vi "Disabled.vi"(7 "Robot Mode":T2, 10 "Match Info":T1={"Autonomous Elapsed Seconds"=0.0, "TeleOp Elapsed Seconds"=0.0, "Disabled Elapsed Seconds"=0.0, "Visited Autonomous"=FALSE, "Visited TeleOp"=FALSE, "Visited Disabled"=FALSE, "Autonomous Settings"={"Autonomous Style"=enum."Independent", "VI Refnum"=refnum}}, 11 "Call Context":T3) -> ()   [LabVIEW 2012]
doc: "This VI is called each time a disabled packet is received from the DS. It is often used to prepare for the next robot mode, to calibrate sensors, etc."
uses:
  <vilib>/Rock Robotics/WPI/DriverStation/WPI_DriverStationDerivedRobotMode.ctl
  <vilib>/Rock Robotics/WPI/DriverStation/WPI_DriverStationRobotMode2.ctl
  <vilib>/Rock Robotics/WPI/DriverStation/WPI_DriverStationMatch Info.ctl
  Robot Global Data.vi
  <vilib>/Rock Robotics/WPI/Joystick/WPI_JoystickGetSetRefNum.vi
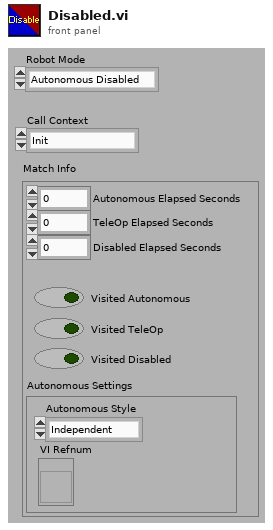
[diagram p1: front panel]
types:
  T1 = typedef "WPI_DriverStationMatch Info.ctl" = cluster{"Autonomous Elapsed Seconds":dbl, "TeleOp Elapsed Seconds":dbl, "Disabled Elapsed Seconds":dbl, "Visited Autonomous":bool, "Visited TeleOp":bool, "Visited Disabled":bool, "Autonomous Settings":cluster{"Autonomous Style":enum16{"Iterative", "Independent"}, "VI Refnum":refnum<vi>}}
  T2 = typedef "WPI_DriverStationRobotMode2.ctl" = enum16{"Autonomous Disabled", "Autonomous Enabled", "Teleop Disabled", "Teleop Enabled", "Timeout", "Finish", "Test Disabled", "Test Enabled"}
  T3 = typedef "WPI_DriverStationDerivedRobotMode.ctl" = enum16{"Init", "Execute", "Stop"}
  T4 = typedef "WPI_JoystickDevRef.ctl" = cluster{"Device":T5}
  T5 = typedef "WPI_JoystickDeviceEnum.ctl" = enum16{"USB 1", "USB 2", "USB 3", "USB 4", "Kinect 1", "Kinect 2"}
  T6 = typedef "WPI_JoystickButtonState.ctl" = cluster{"Button 1":bool, "Button 2":bool, "Button 3":bool, "Button 4":bool, "Button 5":bool, "Button 6":bool, "Button 7":bool, "Button 8":bool, "Button 9":bool, "Button 10":bool, "Button 11":bool, "Button 12":bool}
  T7 = cluster{"Setpoint 1":dbl, "Setpoint 2":dbl, "Setpoint 3":dbl, "Setpoint 4":dbl, "RotLow":dbl, "RotHigh":dbl, "ExtLow":dbl, "ExtHigh":dbl}
  T8 = cluster{"FlipperLeftUp":dbl, "FlipperLeftDown":dbl, "FlipperRightUp":dbl, "FlipperRightDown":dbl, "KickerLeftBack":dbl, "KickerLeftForward":dbl, "KickerRightBack":dbl, "KickerRightForward":dbl}
  T9 = typedef "WPI_MotorControlDeviceRef.ctl" = cluster{"DeviceStatus":errorcluster, "Type":enum16{"PWM", "CAN"}, "PWM":cluster{"Digital Module":T10, "PWM Channel":T11, "DeadBand":T12}, "CAN":cluster{"Device Number":u8, "Control Mode":T13, "Semaphore":T14, "Max Vout":dbl}, "Invert":bool, "TransformRef":T15, "InvTransformRef":T15}
  T10 = typedef "FPGA_TypedefDigitalModule.ctl" = enum16{"Digital Module 1", "Digital Module 2"}
  T11 = typedef "FPGA_DIOPWMChannel.ctl" = enum8{"PWM 1", "PWM 2", "PWM 3", "PWM 4", "PWM 5", "PWM 6", "PWM 7", "PWM 8", "PWM 9", "PWM 10", "Invalid"}
  T12 = typedef "WPI_PWMDeadband.ctl" = cluster{"Name":string, "maxPositivePwm":i32, "minPositivePwm":i32, "centerPwm":i32, "maxNegativePwm":i32, "minNegativePwm":i32, "angularRange":u16}
  T13 = typedef "WPI_CANJaguar_ControlMode.ctl" = enum8{"Percent VBus", "Current", "Speed", "Position", "Voltage"}
  T14 = typedef "Semaphore RefNum" = refnum<k1>
  T15 = typedef "WPI_PWMTransform_ConPane.ctl" = refnum<vi>
  T16 = typedef "WPI_ServoDeviceRef.ctl" = cluster{"DeviceStatus":errorcluster, "Digital Module":T10, "PWM Channel":T11, "DeadBand":T12}
  T17 = cluster{"Right Servo High":dbl, "Right Servo Mid":dbl, "Right Servo Low":dbl, "Left Servo High":dbl, "Left Servo Mid":dbl, "Left Servo Low":dbl}
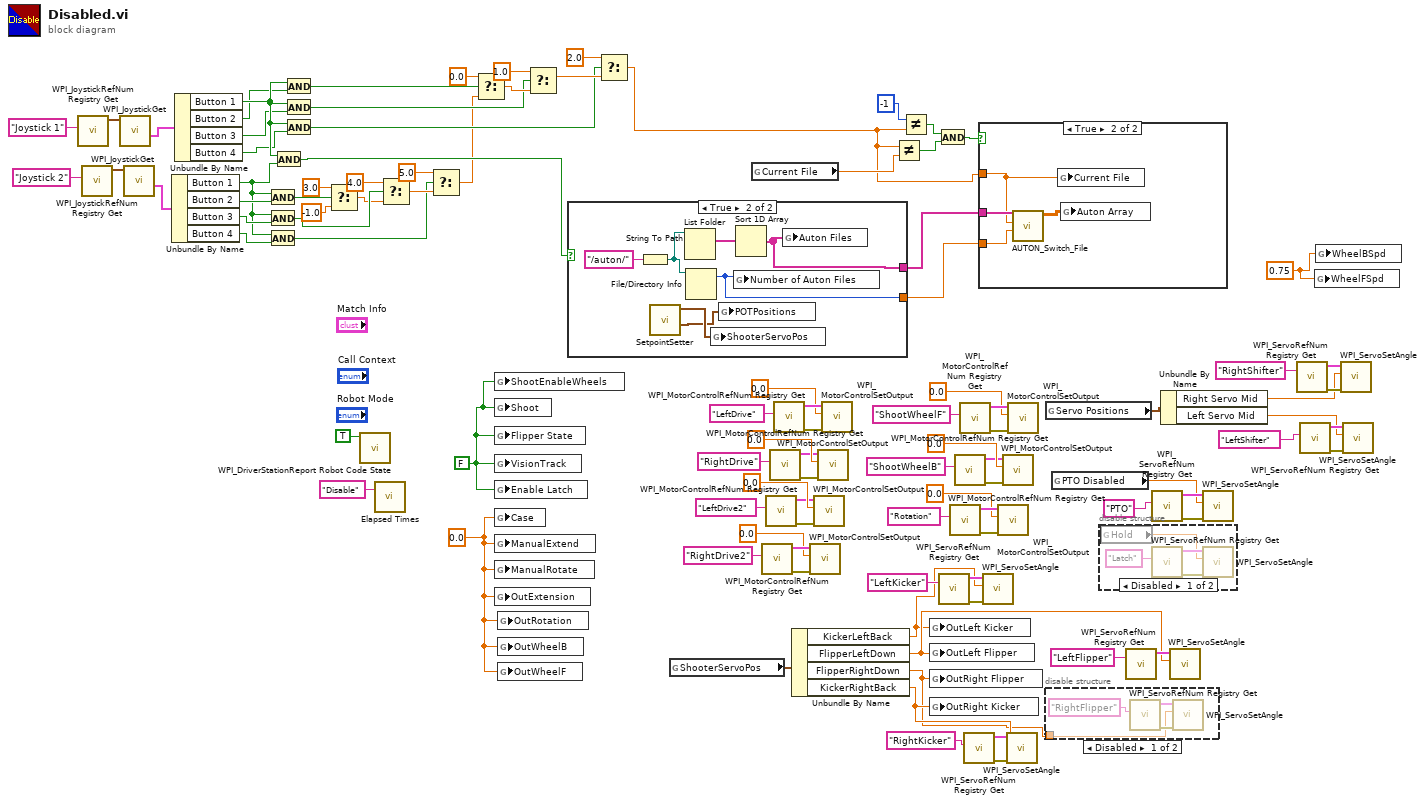
[diagram p0: block diagram]
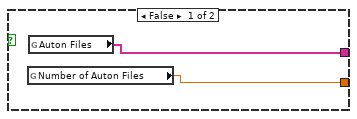
[diagram p5: hidden frame]
diagram:
  w35 = 0.75 ("Case")
  w54 = 0.0 ("Case")
  w55 = FALSE ("Enable Latch")
  n1 = call <vilib>:"WPI_JoystickRefNum Registry Get.vi"("refnum name"="Joystick 1") -> ("JoystickDevRef"=w33:T4)  [unwired: 9 in, 1 out]
  n2 = call <vilib>:"WPI_JoystickRefNum Registry Get.vi"("refnum name"="Joystick 2") -> ("JoystickDevRef"=w31:T4)  [unwired: 9 in, 1 out]
  n3 = call <vilib>:"WPI_JoystickGet.vi"("JoystickDevRef"=w33) -> ("Buttons"=w29:T6)  [unwired: 4 in, 2 out]
  n4 = call <vilib>:"WPI_JoystickGet.vi"("JoystickDevRef"=w31) -> ("Buttons"=w30:T6)  [unwired: 4 in, 2 out]
  n5 = Unbundle By Name(w30) -> ("Button 1"=w26:bool, "Button 2"=w28:bool, "Button 3"=w27:bool, "Button 4"=w25:bool)
  n6 = Unbundle By Name(w29) -> ("Button 1"=w7:bool, "Button 2"=w6:bool, "Button 3"=w5:bool, "Button 4"=w4:bool)
  n7 = And(x=w26, y=w28) -> (x .and. y?=w24:bool)
  n8 = And(x=w26, y=w27) -> (x .and. y?=w21:bool)
  n9 = And(x=w26, y=w25) -> (x .and. y?=w15:bool)
  n10 = And(x=w7, y=w26) -> (x .and. y?=w17:bool)
  n11 = And(x=w7, y=w6) -> (x .and. y?=w8:bool)
  n12 = And(x=w7, y=w5) -> (x .and. y?=w10:bool)
  n13 = And(x=w7, y=w4) -> (x .and. y?=w3:bool)
  n14 = Select(t=3.0, s=w24, f=-1.0) -> (s? t:f=w20:dbl)
  n15 = call <vilib>:"WPI_DriverStationReport Robot Code State.vi"("Disabled"=TRUE ("Autonomous")) -> ()  [unwired: 10 in, 1 out]
  n16 = call "Elapsed Times.vi"("Call Name"="Disable") -> ()  [unwired: 2 in, 1 out]
  n17 = Select(t=4.0, s=w21, f=w20) -> (s? t:f=w18:dbl)
  n18 = Select(t=5.0, s=w15, f=w18) -> (s? t:f=w2:dbl)
  n19 = Select(t=0.0, s=w8, f=w2) -> (s? t:f=w11:dbl)
  n20 = global write "Robot Global Data.vi" "ShootEnableWheels"(w55) -> ()
  n21 = global write "Robot Global Data.vi" "Shoot"(w55) -> ()
  n22 = global write "Robot Global Data.vi" "Flipper State"(w55) -> ()
  n23 = global write "Robot Global Data.vi" "VisionTrack"(w55) -> ()
  n24 = global write "Robot Global Data.vi" "Enable Latch"(w55) -> ()
  n25 = global write "Robot Global Data.vi" "Case"(w54) -> ()
  n26 = global write "Robot Global Data.vi" "ManualExtend"(w54) -> ()
  n27 = global write "Robot Global Data.vi" "ManualRotate"(w54) -> ()
  n28 = global write "Robot Global Data.vi" "OutExtension"(w54) -> ()
  n29 = global write "Robot Global Data.vi" "OutRotation"(w54) -> ()
  n30 = global write "Robot Global Data.vi" "OutWheelB"(w54) -> ()
  n31 = global write "Robot Global Data.vi" "OutWheelF"(w54) -> ()
  n32 = Select(t=1.0, s=w10, f=w11) -> (s? t:f=w13:dbl)
  n33 = case shown="True" w17 {
    tunnel: [w101 w106] -> w90
    tunnel: [w102 w105] -> w85
    frame False {
      n34 = global read "Robot Global Data.vi" "Number of Auton Files"() -> (w101:dbl)
      n35 = global read "Robot Global Data.vi" "Auton Files"() -> (w102:string[])
    }
    frame True {
      n36 = String To Path(string="/auton/") -> (path=w108:path)
      n37 = call "SetpointSetter.vi"() -> ("Arm Pos"=w103:T7, "Shooter Servo Pos"=w104:T8)  [unwired: 10 in]
      n38 = List Folder(path=w108) -> (filenames=w107:string[])  [unwired: 3 in, 3 out]
      n39 = File/Directory Info(path=w108) -> (size=w106:i64)  [unwired: 1 in, 6 out]
      n40 = global write "Robot Global Data.vi" "ShooterServoPos"(w104) -> ()
      n41 = global write "Robot Global Data.vi" "POTPositions"(w103) -> ()
      n42 = global write "Robot Global Data.vi" "Number of Auton Files"(w106) -> ()
      n43 = Sort 1D Array(array=w107) -> (sorted array=w105:string[])
      n44 = global write "Robot Global Data.vi" "Auton Files"(w105) -> ()
    }
  }
  n45 = Select(t=2.0, s=w3, f=w13) -> (s? t:f=w1:dbl)
  n46 = global read "Robot Global Data.vi" "ShooterServoPos"() -> (w53:T8)
  n47 = global read "Robot Global Data.vi" "Current File"() -> (w88:dbl)
  n48 = call <vilib>:"WPI_MotorControlRefNum Registry Get.vi"("refnum name"="RightDrive2") -> ("error out"=w71:errorcluster, "MotorControlDevRef"=w70:T9)  [unwired: 9 in]
  n49 = call <vilib>:"WPI_MotorControlRefNum Registry Get.vi"("refnum name"="LeftDrive2") -> ("error out"=w64:errorcluster, "MotorControlDevRef"=w65:T9)  [unwired: 9 in]
  n50 = call <vilib>:"WPI_MotorControlRefNum Registry Get.vi"("refnum name"="RightDrive") -> ("error out"=w91:errorcluster, "MotorControlDevRef"=w92:T9)  [unwired: 9 in]
  n51 = call <vilib>:"WPI_MotorControlRefNum Registry Get.vi"("refnum name"="LeftDrive") -> ("error out"=w98:errorcluster, "MotorControlDevRef"=w97:T9)  [unwired: 9 in]
  n52 = Unbundle By Name(w53) -> ("KickerLeftBack"=w50:dbl, "FlipperLeftDown"=w51:dbl, "FlipperRightDown"=w49:dbl, "KickerRightBack"=w52:dbl)
  n53 = call <vilib>:"WPI_MotorControlSetOutput.vi"("error in (no error)"=w71, "Output"=0.0, "MotorControlDevRef"=w70) -> ()  [unwired: 6 in, 3 out]
  n54 = call <vilib>:"WPI_MotorControlSetOutput.vi"("error in (no error)"=w64, "Output"=0.0, "MotorControlDevRef"=w65) -> ()  [unwired: 6 in, 3 out]
  n55 = call <vilib>:"WPI_MotorControlSetOutput.vi"("error in (no error)"=w91, "Output"=0.0, "MotorControlDevRef"=w92) -> ()  [unwired: 6 in, 3 out]
  n56 = call <vilib>:"WPI_MotorControlSetOutput.vi"("error in (no error)"=w98, "Output"=0.0, "MotorControlDevRef"=w97) -> ()  [unwired: 6 in, 3 out]
  n57 = Not Equal?(x=w1, y=w88) -> (x != y?=w86:bool)
  n58 = Not Equal?(x=-1, y=w1) -> (x != y?=w87:bool)
  n59 = global write "Robot Global Data.vi" "OutLeft Kicker"(w50) -> ()
  n60 = global write "Robot Global Data.vi" "OutLeft Flipper"(w51) -> ()
  n61 = global write "Robot Global Data.vi" "OutRight Flipper"(w49) -> ()
  n62 = global write "Robot Global Data.vi" "OutRight Kicker"(w52) -> ()
  n63 = And(x=w87, y=w86) -> (x .and. y?=w84:bool)
  n64 = call <vilib>:"WPI_ServoRefNum Registry Get.vi"("refnum name"="LeftKicker") -> ("error out"=w56:errorcluster, "ServoDeviceRef"=w57:T16)  [unwired: 9 in]
  n65 = call <vilib>:"WPI_MotorControlRefNum Registry Get.vi"("refnum name"="Rotation") -> ("error out"=w75:errorcluster, "MotorControlDevRef"=w74:T9)  [unwired: 9 in]
  n66 = call <vilib>:"WPI_MotorControlRefNum Registry Get.vi"("refnum name"="ShootWheelB") -> ("error out"=w76:errorcluster, "MotorControlDevRef"=w77:T9)  [unwired: 9 in]
  n67 = call <vilib>:"WPI_MotorControlRefNum Registry Get.vi"("refnum name"="ShootWheelF") -> ("error out"=w83:errorcluster, "MotorControlDevRef"=w82:T9)  [unwired: 9 in]
  n68 = call <vilib>:"WPI_ServoRefNum Registry Get.vi"("refnum name"="RightKicker") -> ("error out"=w62:errorcluster, "ServoDeviceRef"=w60:T16)  [unwired: 9 in]
  n69 = case shown="True" w84 {
    tunnel: w85 -> [_ w113]
    tunnel: w90 -> [_ w112]
    tunnel: w1 -> [_ w110]
    frame False {
    }
    frame True {
      n70 = call "AUTON_Switch_File.vi"("Number of Auton Files"=w112, "Auton File"=w110, "Auton Files"=w113) -> ("Auton Array"=w111:dbl[][])  [unwired: 7 in, 1 out]
      n71 = global write "Robot Global Data.vi" "Current File"(w110) -> ()
      n72 = global write "Robot Global Data.vi" "Auton Array"(w111) -> ()
    }
  }
  n73 = call <vilib>:"WPI_ServoSetAngle.vi"("error in (no error)"=w56, "Angle"=w50, "ServoDeviceRef"=w57) -> ()  [unwired: 7 in, 2 out]
  n74 = call <vilib>:"WPI_MotorControlSetOutput.vi"("error in (no error)"=w75, "Output"=0.0, "MotorControlDevRef"=w74) -> ()  [unwired: 6 in, 3 out]
  n75 = call <vilib>:"WPI_MotorControlSetOutput.vi"("error in (no error)"=w76, "Output"=0.0, "MotorControlDevRef"=w77) -> ()  [unwired: 6 in, 3 out]
  n76 = call <vilib>:"WPI_ServoSetAngle.vi"("error in (no error)"=w62, "Angle"=w52, "ServoDeviceRef"=w60) -> ()  [unwired: 7 in, 2 out]
  n77 = call <vilib>:"WPI_MotorControlSetOutput.vi"("error in (no error)"=w83, "Output"=0.0, "MotorControlDevRef"=w82) -> ()  [unwired: 6 in, 3 out]
  n78 = global read "Robot Global Data.vi" "Servo Positions"() -> (w39:T17)
  n79 = disable-structure shown="Disabled" {
    disable-tunnel: w49 -> [w114 _]
    frame Disabled {
      n80 = call <vilib>:"WPI_ServoRefNum Registry Get.vi"("refnum name"="RightFlipper") -> ("error out"=w117:errorcluster, "ServoDeviceRef"=w115:T16)  [unwired: 9 in]
      n81 = call <vilib>:"WPI_ServoSetAngle.vi"("error in (no error)"=w117, "Angle"=w114, "ServoDeviceRef"=w115) -> ()  [unwired: 7 in, 2 out]
    }
    frame Enabled {
    }
  }
  n82 = global read "Robot Global Data.vi" "PTO Disabled"() -> (w36:dbl)
  n83 = disable-structure shown="Disabled" {
    frame Disabled {
      n84 = global read "Robot Global Data.vi" "Hold"() -> (w118:dbl)
      n85 = call <vilib>:"WPI_ServoRefNum Registry Get.vi"("refnum name"="Latch") -> ("error out"=w119:errorcluster, "ServoDeviceRef"=w120:T16)  [unwired: 9 in]
      n86 = call <vilib>:"WPI_ServoSetAngle.vi"("error in (no error)"=w119, "Angle"=w118, "ServoDeviceRef"=w120) -> ()  [unwired: 7 in, 2 out]
    }
    frame Enabled {
    }
  }
  n87 = call <vilib>:"WPI_ServoRefNum Registry Get.vi"("refnum name"="LeftFlipper") -> ("ServoDeviceRef"=w58:T16)  [unwired: 9 in, 1 out]
  n88 = call <vilib>:"WPI_ServoRefNum Registry Get.vi"("refnum name"="PTO") -> ("error out"=w40:errorcluster, "ServoDeviceRef"=w42:T16)  [unwired: 9 in]
  n89 = Unbundle By Name(w39) -> ("Right Servo Mid"=w37:dbl, "Left Servo Mid"=w38:dbl)
  n90 = call <vilib>:"WPI_ServoSetAngle.vi"("Angle"=w51, "ServoDeviceRef"=w58) -> ()  [unwired: 8 in, 2 out]
  n91 = call <vilib>:"WPI_ServoSetAngle.vi"("error in (no error)"=w40, "Angle"=w36, "ServoDeviceRef"=w42) -> ()  [unwired: 7 in, 2 out]
  n92 = call <vilib>:"WPI_ServoRefNum Registry Get.vi"("refnum name"="RightShifter") -> ("error out"=w45:errorcluster, "ServoDeviceRef"=w46:T16)  [unwired: 9 in]
  n93 = call <vilib>:"WPI_ServoRefNum Registry Get.vi"("refnum name"="LeftShifter") -> ("error out"=w47:errorcluster, "ServoDeviceRef"=w48:T16)  [unwired: 9 in]
  n94 = global write "Robot Global Data.vi" "WheelFSpd"(w35) -> ()
  n95 = global write "Robot Global Data.vi" "WheelBSpd"(w35) -> ()
  n96 = call <vilib>:"WPI_ServoSetAngle.vi"("error in (no error)"=w45, "Angle"=w37, "ServoDeviceRef"=w46) -> ()  [unwired: 7 in, 2 out]
  n97 = call <vilib>:"WPI_ServoSetAngle.vi"("error in (no error)"=w47, "Angle"=w38, "ServoDeviceRef"=w48) -> ()  [unwired: 7 in, 2 out]
